vi "HttpClient.vi"(7 "™z²é î‘B?":bool, 8 "error in (no error)":errorcluster caption="错误输入（无错误）", 10 "±í†Î”µ“þ":T1, 11 "HttpClient 输入":refnum<class "Http.lvclass"> caption="DNL_LabVIEW Object in") -> (0 "error out":errorcluster caption="错误输出", 1 "”µ“þ":string, 2 "î‘B":i32, 3 "HttpClient 输出":refnum<class "Http.lvclass"> caption="DNL_LabVIEW Object out", 4 "body":string caption="体部", 6 "headers":string caption="头部")   [LabVIEW 2012, in "Http.lvclass"]
uses:
  Http.lvclass
  HttpData.ctl
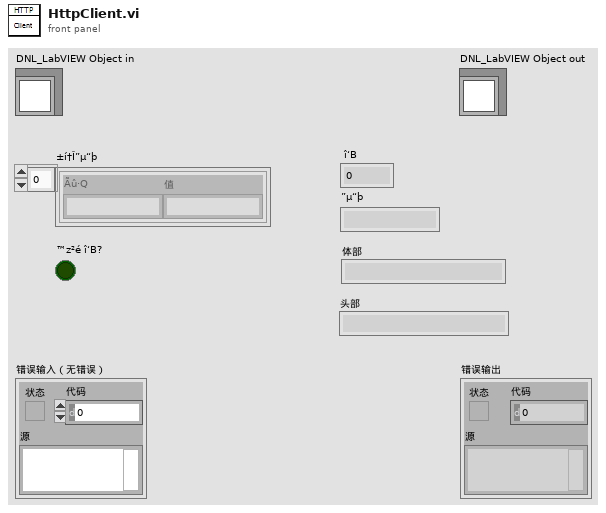
[diagram p1: front panel]
types:
  T1 = typedef "Http.lvclass/HttpData.ctl" = cluster{"Ãû·Q":string, "值":string}[]
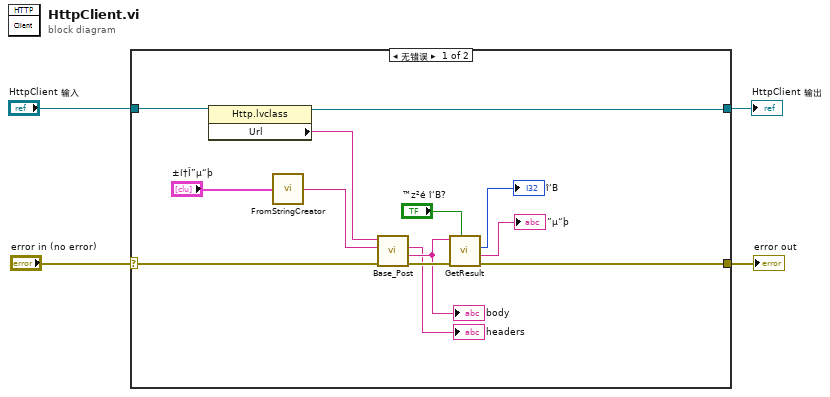
[diagram p0: block diagram]
diagram:
  n1 = case shown="无错误" "error in (no error)" {
    selector: "error in (no error)" -> [w13 w19]
    tunnel: [w11 w19] -> w3
    tunnel: [w9 w18] -> w1
    tunnel: "HttpClient 输入" -> [w16 w18]
    frame No Error {
      n2 = property class="Http.lvclass"(reference=w16) -> (reference out=w9:refnum<class "Http.lvclass">, "Url"=w15:string)  [unwired: 1 in, 1 out]
      n3 = call "FromStringCreator.vi"("±í†Î”µ“þ"="±í†Î”µ“þ") -> ("表單字串"=w14:string)  [unwired: 4 in]
      n4 = call "Base_Post.vi"("error in (no error)"=w13, "buffer"=w14, "url"=w15) -> ("error out"=w12:errorcluster, "body"=w10:string, "headers"=→"headers":string)  [unwired: 6 in]
      "body" <- w10
      n5 = call "GetResult.vi"("HttpBuff"=w10, "error in (no error)"=w12, "™z²é î‘B?"="™z²é î‘B?") -> ("î‘B"=→"î‘B":i32, "”µ“þ"=→"”µ“þ":string, "error out"=w11:errorcluster)  [unwired: 5 in]
    }
    frame Error {
    }
  }
  "error out" <- w3
  "HttpClient 输出" <- w1
